vi "Save Trigger Event.vi"(4 "Consumer Synch\nSemaphore":T1, 6 "Event Queue":refnum<queue>, 8 "error in (no error)":errorcluster, 10 "DAQ Fetch Queue":refnum<queue>, 11 "refnum in":refnum<file>) -> (0 "error out":errorcluster, 1 "Trigger Event":dbl[][](array[numeric]), 2 "DAQ Fetch Queue Out":refnum<queue>, 3 "refnum out":refnum<file>)   [LabVIEW 2012]
panel:
  out "# Triggers":i32=3
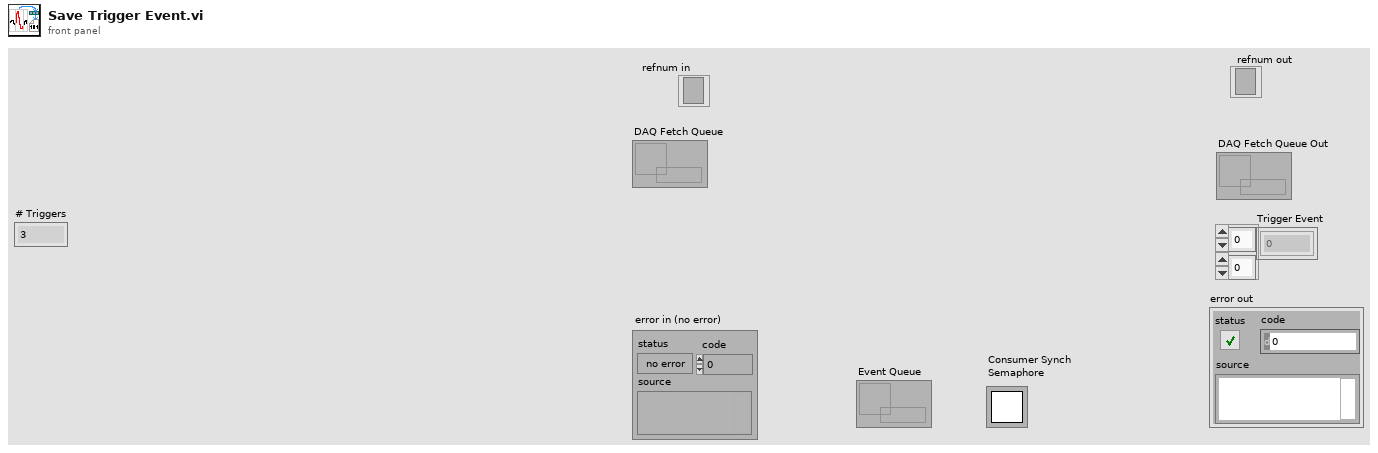
[diagram p1: front panel]
types:
  T1 = typedef "Semaphore RefNum" = refnum<k1>
  T2 = enum16{"big-endian, network order", "native, host order", "little-endian"}
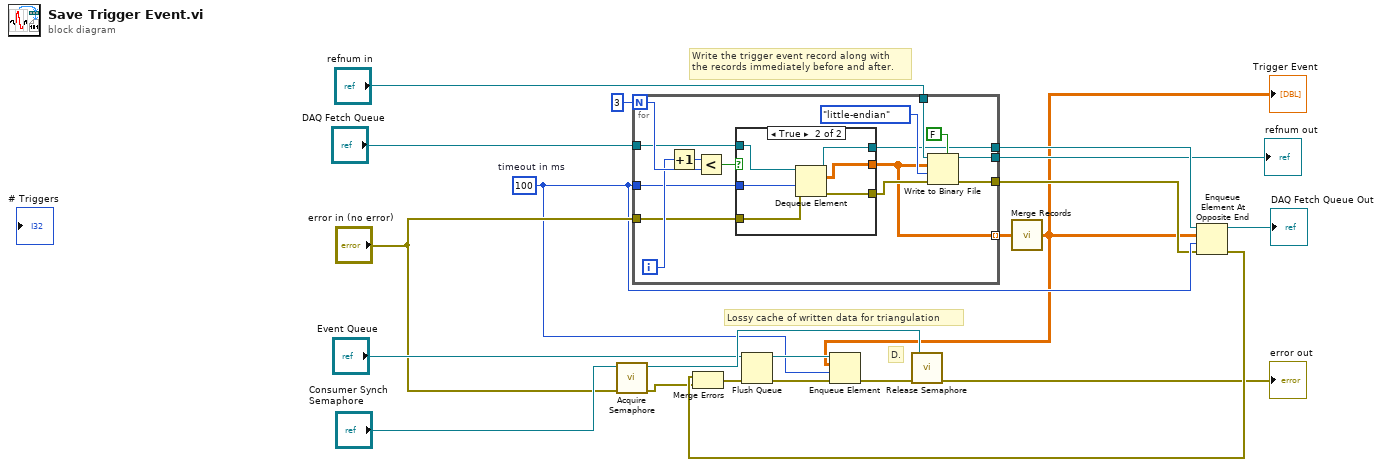
[diagram p0: block diagram]
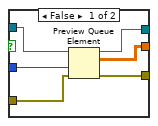
[diagram p2: hidden frame]
diagram:
  w8 = 100  # timeout in ms
  # "Lossy cache of written data for triangulation"
  # "D."
  # "Write the trigger event record along with\nthe records immediately before and after."
  n1 = call <vilib>:"Acquire Semaphore.vi"("error in (no error)"="error in (no error)", "semaphore"="Consumer Synch\nSemaphore") -> ("error out"=w11:errorcluster, "semaphore out"=w20:T1)  [unwired: 3 in, 1 out]
  n2 = for {
    N: 3 -> [w33]
    tunnel: "DAQ Fetch Queue" -> [w30]
    tunnel: w8 -> [w29]
    tunnel: "error in (no error)" -> [w28]
    tunnel: [w27] -> w6
    tunnel: [w26] -> w3
    tunnel: "refnum in" -> [w25]
    tunnel: [w24] -> w2 mode=indexing
    tunnel: [w22] -> w5
    i -> [w31]
    n3 = Increment(x=w31) -> (x+1=w32:i32)
    n4 = Less?(x=w32, y=w33) -> (x < y?=w34:bool)
    n5 = case shown="True" w34 {
      tunnel: [w40 w48] -> w24
      tunnel: [w41 w47] -> w36
      tunnel: w30 -> [w42 w46]
      tunnel: w29 -> [w39 w45]
      tunnel: w28 -> [w38 w43]
      tunnel: [w37 w44] -> w22
      frame False {
        n6 = Preview Queue Element(queue=w42, timeout in ms (-1)=w39, error in (no error)=w38) -> (queue out=w37:refnum<queue>, element=w40:dbl[][], error out=w41:errorcluster)  [unwired: 1 out]
      }
      frame True {
        n7 = Dequeue Element(queue=w46, timeout in ms (-1)=w45, error in (no error)=w43) -> (queue out=w44:refnum<queue>, element=w48:dbl[][], error out=w47:errorcluster)  [unwired: 1 out]
      }
    }
    n8 = Write to Binary File(file (use dialog)=w25, data=w24, error in=w36, 5:FALSE ("prepend array or string size? (T)"), 9:T2."little-endian" ("byte order (0:big-endian, network order)")) -> (refnum out=w26:refnum<file>, error out=w27:errorcluster)  [unwired: 1 in, 1 out]
  }
  "refnum out" <- w3
  n9 = call "Merge Records.vi"("Records"=w2) -> ("Channel Data"=w1:dbl[][])  [unwired: 4 in]
  "Trigger Event" <- w1
  n10 = Enqueue Element At Opposite End(queue=w5, element=w1, timeout in ms (-1)=w8, error in (no error)=w6) -> (queue out=→"DAQ Fetch Queue Out":refnum<queue>, error out=w18:errorcluster)  [unwired: 1 out]
  n11 = Merge Errors(w18, w11) -> (w19:errorcluster)
  n12 = Flush Queue(queue="Event Queue", error in (no error)=w19) -> (queue out=w9:refnum<queue>, error out=w10:errorcluster)  [unwired: 1 out]
  n13 = Enqueue Element(queue=w9, element=w1, timeout in ms (-1)=w8, error in (no error)=w10) -> (error out=w7:errorcluster)  [unwired: 2 out]
  n14 = call <vilib>:"Release Semaphore.vi"("error in (no error)"=w7, "semaphore"=w20) -> ("error out"=→"error out":errorcluster)  [unwired: 4 in, 1 out]
